vi "SmartSEM Remote API detectors.vi"(7 "Iterations":u32=3, 8 "error in":errorcluster, 9 "Det B Type":string, 10 "Det A Type":string, 11 "Api":refnum<k7>(container)) -> (0 "error out":errorcluster, 3 "Api out":refnum<k7>)   [LabVIEW 2018]
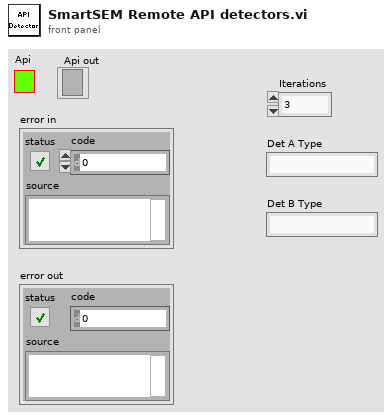
[diagram p1: front panel]
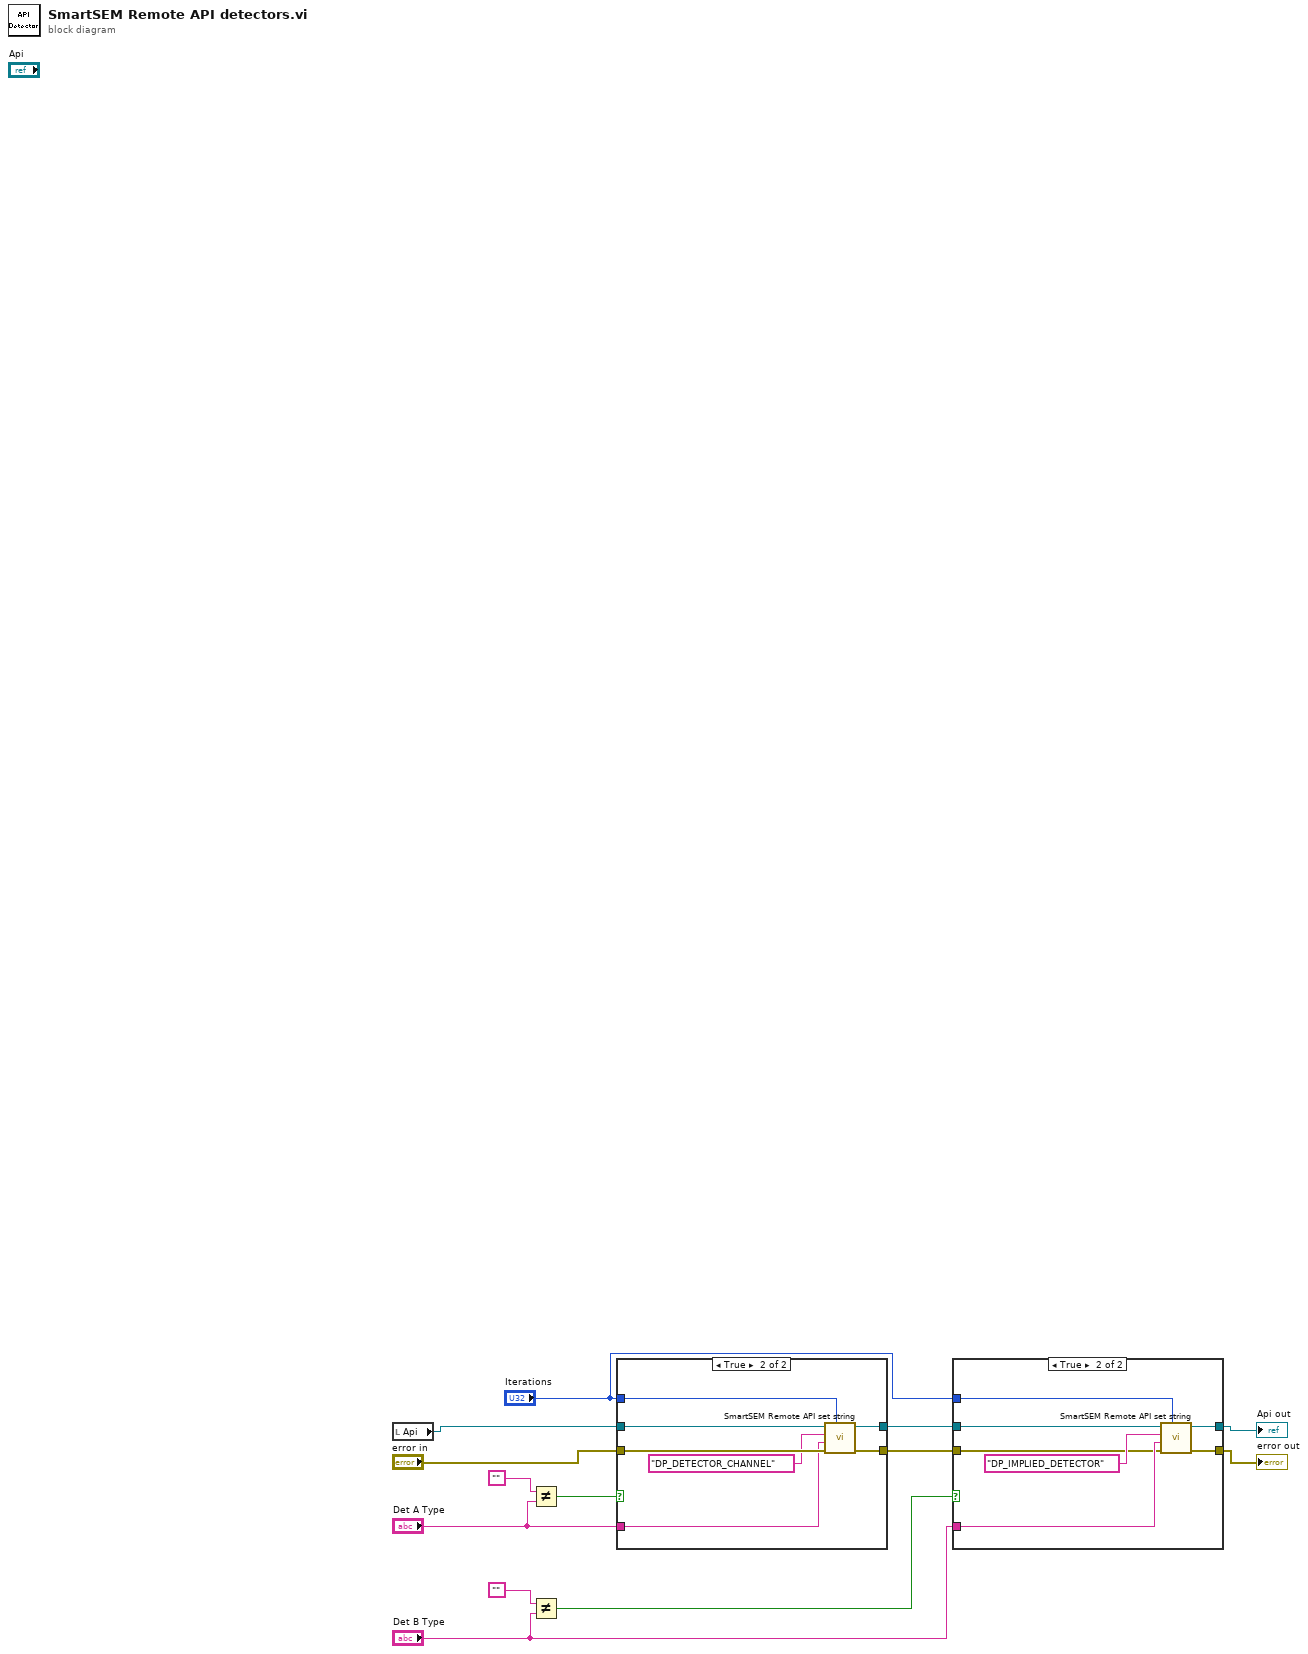
[diagram p0: block diagram]
diagram:
  n1 = local read "Api"() -> (w8:refnum<k7>)
  n2 = Not Equal?(x="", y="Det A Type") -> (x != y?=w11:bool)
  n3 = Not Equal?(x="", y="Det B Type") -> (x != y?=w6:bool)
  n4 = case shown="True" w11 {
    tunnel: w8 -> [w15 w22]
    tunnel: "error in" -> [w14 w21]
    tunnel: "Det A Type" -> [_ w20]
    tunnel: [w15 w17] -> w3
    tunnel: [w14 w16] -> w4
    tunnel: "Iterations" -> [_ w18]
    frame False {
    }
    frame True {
      n5 = call "SmartSEM Remote API set string.vi"("Iterations"=w18, "error in"=w21, "vValue"=w20, "lpszParam"="DP_DETECTOR_CHANNEL" ("lpszCommand"), "Api"=w22) -> ("error out"=w16:errorcluster, "Api out"=w17:refnum<k7>)  [unwired: 5 in]
    }
  }
  n6 = case shown="True" w6 {
    tunnel: w3 -> [w24 w26]
    tunnel: w4 -> [w23 w25]
    tunnel: "Det B Type" -> [_ w31]
    tunnel: [w24 w29] -> w2
    tunnel: [w23 w28] -> w1
    tunnel: "Iterations" -> [_ w30]
    frame False {
    }
    frame True {
      n7 = call "SmartSEM Remote API set string.vi"("Iterations"=w30, "error in"=w25, "vValue"=w31, "lpszParam"="DP_IMPLIED_DETECTOR" ("lpszCommand"), "Api"=w26) -> ("error out"=w28:errorcluster, "Api out"=w29:refnum<k7>)  [unwired: 5 in]
    }
  }
  "Api out" <- w2
  "error out" <- w1
